vi "SubVI_CloseCamera.vi"(11 "ErrorIn":errorcluster) -> (0 "u8Error":u8, 3 "ErrorOut":errorcluster)   [LabVIEW 2013]
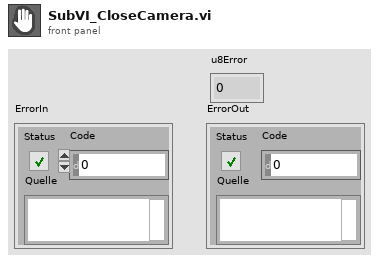
[diagram p1: front panel]
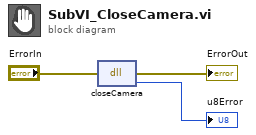
[diagram p0: block diagram]
diagram:
  n1 = dll-call lib="PTH1abs CUsers1000len-bimDesktop&Lieferung_LabView_Interface_11.11.2015Einrichten fÃ¼r - EndkundenDatenTesto_v2013VIlabview_cwrapper_1_0_0.dll" fn="closeCamera"(error in="ErrorIn") -> (error out=→"ErrorOut":errorcluster, "u8Error"=→"u8Error":u8)  [unwired: 2 in, 1 out]
